vi "Get AO Channel Count.vi"(3 "DAQ []":T1 {"AI.Coupling" items=["AC"=10045, "DC"=10050, "GND"=10066]}) -> (1 "# AO channels":i32)   [LabVIEW 2019, in "Instrument.Lockin.lvlib" / "Instrument UI.Lockin.lvclass"]
uses:
  Instrument UI.Lockin.lvclass
  Instrument.DAQ/Typedefs/DAQ.Configuration--Cluster--Array.ctl
  Instrument.DAQ/Typedefs/DAQ.Configuration--Cluster.ctl
  Instrument.DAQ/Typedefs/DAQ.Config.AO.Range--enum.ctl
  Instrument.DAQ/Typedefs/DAQ.Config.AI.Range--enum.ctl
  Instrument.DAQ/Typedefs/DAQ.Config.AI.Coupling--enum.ctl
  Instrument.DAQ/Instrument.DAQ.lvclass
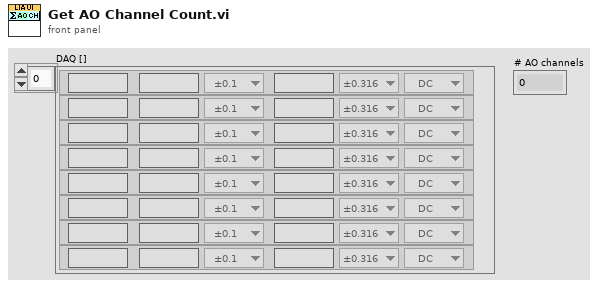
[diagram p1: front panel]
types:
  T1 = typedef "Instrument.Lockin.lvlib/Instrument.DAQ.lvclass/DAQ.Configuration--Cluster--Array.ctl" = T2[]
  T2 = typedef "Instrument.Lockin.lvlib/Instrument.DAQ.lvclass/DAQ.Configuration--Cluster.ctl" = cluster{"Device":string, "AO.Ch":string, "AO.Range":T3, "AI.Ch":string, "AI.Range":T4, "AI.Coupling":T5}
  T3 = typedef "Instrument.Lockin.lvlib/Instrument.DAQ.lvclass/DAQ.Config.AO.Range--enum.ctl" = enum16{"±0.1", "±1.0", "±10.0"}
  T4 = typedef "Instrument.Lockin.lvlib/Instrument.DAQ.lvclass/DAQ.Config.AI.Range--enum.ctl" = enum16{"±0.316", "±1.00", "±3.16", "±10.0", "±31.6", "±42.4"}
  T5 = typedef "Instrument.Lockin.lvlib/Instrument.DAQ.lvclass/DAQ.Config.AI.Coupling--enum.ctl" = u16
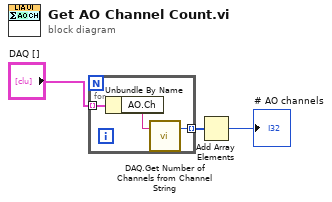
[diagram p0: block diagram]
diagram:
  n1 = for {
    tunnel: "DAQ []" -> [w6] mode=indexing
    tunnel: [w5] -> w1 mode=indexing
    n2 = Unbundle By Name(w6) -> ("AO.Ch"=w4:string)
    n3 = call "DAQ.Get Number of Channels from Channel String.vi"("Channels String"=w4) -> ("# channels"=w5:i32)  [unwired: 2 in]
  }
  n4 = Add Array Elements(numeric array=w1) -> (sum=→"# AO channels":i32)
